vi "Speaker-Init.vi"(7 "Device reference":refnum<vi>, 8 "error in (no error)":errorcluster, 10 "OutputRequest event ref":T1, 11 "InputData reference":refnum<vi>) -> (0 "error out":errorcluster, 2 "OutputRequest (dup)":T1, 3 "InputData (dup)":refnum<vi>)   [LabVIEW 2015]
doc: "Initializes a Speaker object.\n\nInputData reference: create reference from Main VI\nOutputRequest event ref: get this from Rack-Init\nDoor reference: which door to initialize?\n\nThe outputs are just duplicates to make it easier to call a bunch of Device-Init functions."
uses:
  Rack/Typedefs/OutputRequest refnum.ctl
  Rack/Typedefs/OutputRequest.ctl
  Rack/Typedefs/InputData cluster.ctl
  Rack/Methods/Port drivers/DigitalInput-DataCluster.ctl
  Typedefs/Speaker.ctl
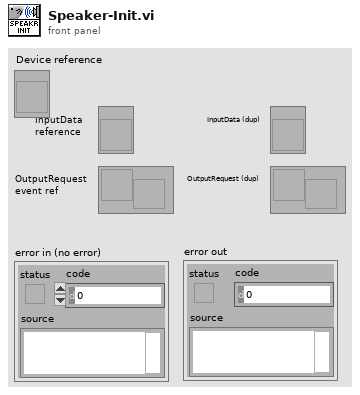
[diagram p1: front panel]
types:
  T1 = typedef "OutputRequest refnum.ctl" = refnum<user-event>
  T2 = typedef "Speaker.ctl" = cluster{"Settings":cluster{"Portname":string, "Index":i32, "Timestamp portname":string}, "OutputRequest event ref":T1, "InputData reference":refnum<vi>}
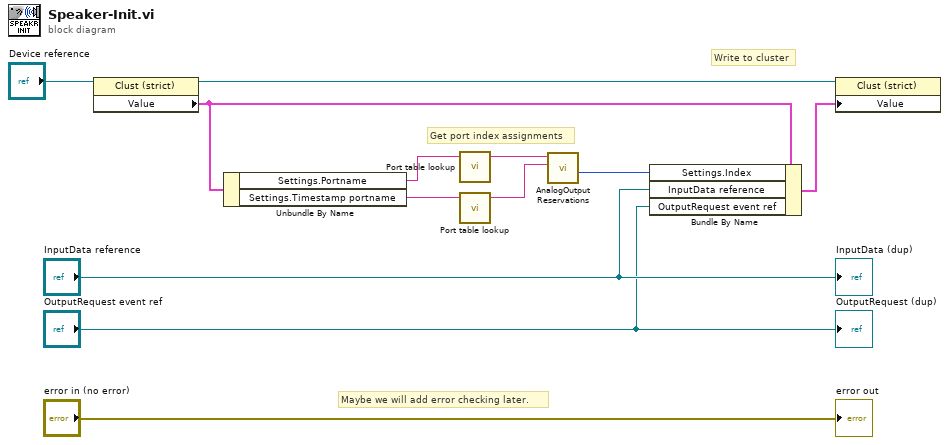
[diagram p0: block diagram]
diagram:
  # "Maybe we will add error checking later."
  # "Write to cluster"
  # "Get port index assignments"
  n1 = property class="Clust (strict)"(reference="Device reference") -> (reference out=w12:refnum<vi>, "Value"=w9:T2)  [unwired: 1 in, 1 out]
  n2 = Unbundle By Name(w9) -> ("Settings.Portname"=w7:string, "Settings.Timestamp portname"=w5:string)
  n3 = call "Port table lookup.vi"("Port name"=w7) -> ("Line"=w10:tag)  [unwired: 3 in, 1 out]
  n4 = call "Port table lookup.vi"("Port name"=w5) -> ("Line"=w4:tag)  [unwired: 3 in, 1 out]
  n5 = call "AnalogOutput Reservations.vi"("Timestamp line"=w4, "Line"=w10) -> ("Index assigned"=w8:i32)  [unwired: 2 in, 3 out]
  n6 = Bundle By Name(cluster=w9, "Settings.Index"=w8, "InputData reference"="InputData reference", "OutputRequest event ref"="OutputRequest event ref") -> (w11:T2)
  n7 = property class="Clust (strict)"(reference=w12, "Value"=w11) -> ()  [unwired: 1 in, 2 out]
  "error out" <- "error in (no error)"
  "OutputRequest (dup)" <- "OutputRequest event ref"
  "InputData (dup)" <- "InputData reference"
